vi "ReportEnd.vi"(6 "文件重命名":bool, 7 "产品型号":string, 8 "error in (no error)":errorcluster caption="错误输入（无错误）", 10 "文件名称":string, 11 "report in":refnum<class "NI_report.lvclass"> caption="报表输入") -> (0 "error out":errorcluster caption="错误输出")   [LabVIEW 2020]
uses:
  <vilib>/Utility/NIReport.llb/NI_report.lvclass
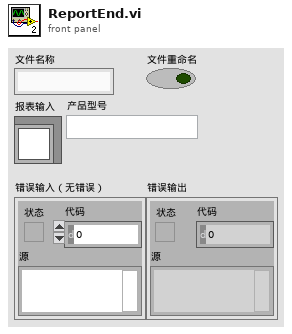
[diagram p1: front panel]
types:
  T1 = cluster{"Italic":enum16{"Italic Unchanged", "Italic On", "Italic Off"}, "Strike Through":enum16{"Strike Through Unchanged", "Strike Through On", "Strike Through Off"}, "Underline":enum16{"Underline Unchanged", "Underline On", "Underline Off"}, "Bold":enum16{"Bold Unchanged", "Bold On", "Bold Off"}}
  T2 = cluster{"Charset (-1)":i16, "Weight (-1)":i16, "Name":string, "Size":string}
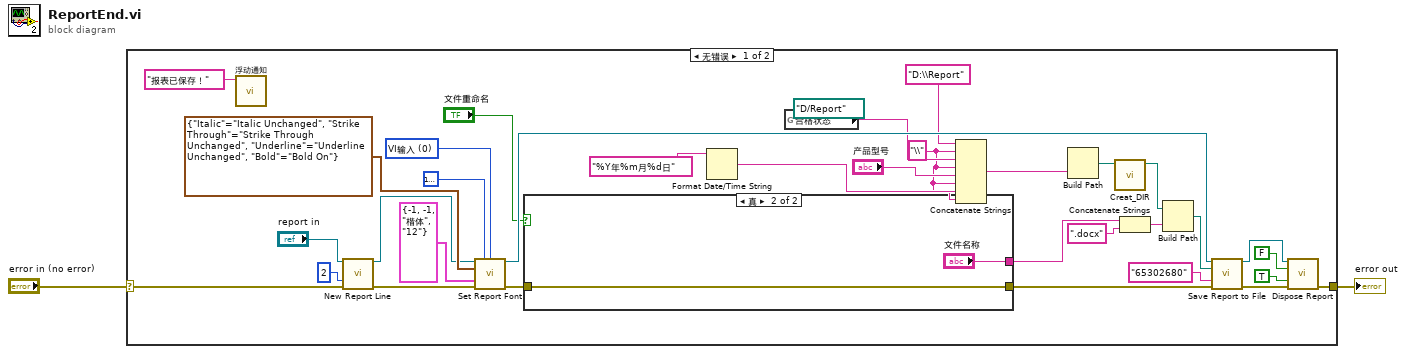
[diagram p0: block diagram]
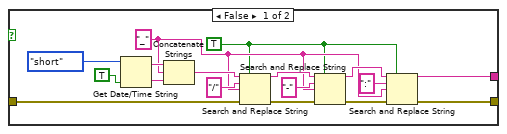
[diagram p2: hidden frame]
diagram:
  n1 = case shown="无错误" "error in (no error)" {
    selector: "error in (no error)" -> [w20 w55]
    tunnel: [w19 w55] -> w1
    frame No Error {
      w4 = "\\"
      w30 = u16 0 items=["VI输入", "字体对话框"] ("font settings source")
      (unwired) path "D:/Report" ("report file path")
      n2 = call "浮动通知.vi"("通知内容"="报表已保存！" ("Status")) -> ()  [unwired: 11 in]
      n3 = call-dynamic "New Report Line.vi"("report in"="report in", "number of lines (1)"=2, "error in (no error)"=w20) -> ("report out"=w27:refnum<class "NI_report.lvclass">, "error out"=w26:errorcluster)  [unwired: 11 in]
      n4 = call-dynamic "Set Report Font.vi"("report in"=w27, "text color (unchanged)"=u32 16777224, "font settings source (VI Inputs)"=w30, "text options"=T1 {"Italic"=enum."Italic Unchanged", "Strike Through"=enum."Strike Through Unchanged", "Underline"=enum."Underline Unchanged", "Bold"=enum."Bold On"}, "font settings"=T2 {"Charset (-1)"=-1, "Weight (-1)"=-1, "Name"="楷体", "Size"="12"}, "error in (no error)"=w26) -> ("report out"=w23:refnum<class "NI_report.lvclass">, "error out"=w22:errorcluster)  [unwired: 7 in, 1 out]
      n5 = case shown="真" "文件重命名" {
        tunnel: [w47 "文件名称"] -> w17
        tunnel: w22 -> [w39 w54]
        tunnel: [w36 w54] -> w21
        frame False {
          w41 = TRUE ("替换全部？(F)")
          w42 = "_" ("替换字符串(\"\")")
          n6 = Get Date/Time String(date format (0)=enum16{"short", "long", "abbreviated"}."short" ("日期格式(0)"), want seconds? (F)=TRUE ("需要秒？(F)")) -> (date string=w52:string, time string=w48:string)  [unwired: 1 in]
          n7 = Concatenate Strings(w52, w42, w48) -> (w45:string)
          n8 = Search and Replace String(replace all?=w41, input string=w45, search string="/" ("搜索字符串"), replace string=w42, error in=w39) -> (result string=w44:string, error out=w38:errorcluster)  [unwired: 3 in, 2 out]
          n9 = Search and Replace String(replace all?=w41, input string=w44, search string="-" ("搜索字符串"), replace string=w42, error in=w38) -> (result string=w50:string, error out=w37:errorcluster)  [unwired: 3 in, 2 out]
          n10 = Search and Replace String(replace all?=w41, input string=w50, search string=":" ("搜索字符串"), replace string=w42, error in=w37) -> (result string=w47:string, error out=w36:errorcluster)  [unwired: 3 in, 2 out]
        }
        frame True {
        }
      }
      n11 = Format Date/Time String(time format string (%c)="%Y年%m月%d日" ("时间格式字符串(%c)")) -> (date/time string=w6:string)  [unwired: 2 in]
      n12 = global read "检测结果.vi" "合格状态"() -> (w7:string)
      n13 = Concatenate Strings("D:\\Report", w4, w7, w4, "产品型号", w4, w6, w4) -> (w5:string)
      n14 = Build Path(name or relative path=w5) -> (appended path=w12:path)  [unwired: 1 in]
      n15 = call "Creat_DIR.vi"("path"=w12) -> ("created path"=w11:path)  [unwired: 10 in]
      n16 = Concatenate Strings(w17, ".docx" ("字符串")) -> (w16:string)
      n17 = Build Path(base path=w11, name or relative path=w16) -> (appended path=w10:path)
      n18 = call-dynamic "Save Report to File.vi"("report in"=w23, "report file path"=w10, "password (\"\")"="65302680" ("password (\"\")"), "error in (no error)"=w21) -> ("report out"=w35:refnum<class "NI_report.lvclass">, "error out"=w34:errorcluster)  [unwired: 10 in]
      n19 = call-dynamic "Dispose Report.vi"("report in"=w35, "wait until printing completed? (T)"=FALSE, "save changes? (F)"=TRUE, "error in (no error)"=w34) -> ("error out"=w19:errorcluster)  [unwired: 11 in]
    }
    frame Error {
    }
  }
  "error out" <- w1
